vi "Finish.vi"   [LabVIEW 2014]
doc: "This VI is called just before exiting. It is expected to close I/O refnum, save collected data, etc."
uses:
  <vilib>/Rock Robotics/WPI/Joystick/WPI_JoystickGetSetRefNum.vi
  <vilib>/Rock Robotics/WPI/RobotDrive/WPI_RobotDriveGetSetRefNum.vi
types:
  T1 = typedef "WPI_JoystickDevRef.ctl" = cluster{"Device":T2}
  T2 = typedef "WPI_JoystickDeviceEnum.ctl" = enum16{"USB 0", "USB 1", "USB 2", "USB 3", "USB 4", "USB 5"}
  T3 = typedef "WPI_RobotDriveDevRef.ctl" = cluster{"DevStatus":errorcluster, "Motors[]":T4[], "Square Inputs":bool, "Max Output":dbl}
  T4 = typedef "WPI_MotorControlDeviceRef.ctl" = cluster{"DeviceStatus":errorcluster, "Type":T5, "PWM":cluster{"Controller":T6, "PWM Channel":T7, "DeadBand":T8}, "CAN":cluster{"Device Number":u8, "Control Mode":T9, "Semaphore":T10, "Max Vout":dbl, "TalonSRX Control Mode":T11}, "Invert":bool, "TransformRef":T12, "InvTransformRef":T12}
  T5 = typedef "WPI_MotorControlType.ctl" = enum16{"PWM", "CAN", "CANTalonSRX"}
  T6 = typedef "FPGA_TypedefDigitalModule.ctl" = enum16{"Controller 1"}
  T7 = typedef "FPGA_DIOPWMChannel.ctl" = enum8{"PWM 0", "PWM 1", "PWM 2", "PWM 3", "PWM 4", "PWM 5", "PWM 6", "PWM 7", "PWM 8", "PWM 9", "PWM MXP 0", "PWM MXP 1", "PWM MXP 2", "PWM MXP 3", "PWM MXP 4", "PWM MXP 5", "PWM MXP 6", "PWM MXP 7", "PWM MXP 8", "PWM MXP 9", "Invalid"}
  T8 = typedef "WPI_PWMDeadband.ctl" = cluster{"Name":string, "maxPositivePwm":i32, "minPositivePwm":i32, "centerPwm":i32, "maxNegativePwm":i32, "minNegativePwm":i32, "angularRange":u16}
  T9 = typedef "WPI_CANJaguar_ControlMode.ctl" = enum8{"Percent VBus", "Current", "Speed", "Position", "Voltage"}
  T10 = typedef "Semaphore RefNum" = refnum<k1>
  T11 = typedef "WPI_CANTalonSRX_APIControlMode.ctl" = enum8{"Percent VBus", "Speed", "Position", "Slave", "Unchanged / Invalid"}
  T12 = typedef "WPI_PWMTransform_ConPane.ctl" = refnum<vi>
  T13 = typedef "WPI_SolenoidDevRef.ctl" = cluster{"DevStatus":errorcluster, "Pneumatics Control Module":u8, "Forward Solenoid Channel":T14, "Reverse Solenoid Channel":T14}
  T14 = typedef "WPI_SolenoidChannel.ctl" = enum8{"Solenoid 0", "Solenoid 1", "Solenoid 2", "Solenoid 3", "Solenoid 4", "Solenoid 5", "Solenoid 6", "Solenoid 7", "Invalid"}
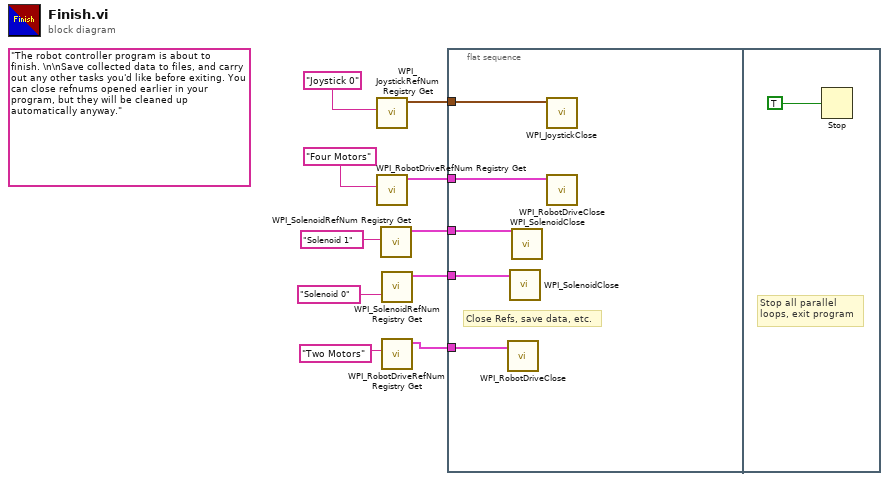
[diagram p0: block diagram]
diagram:
  (unwired) "The robot controller program is about to finish. \n\nSave collected data to files, and carry out any other tasks you'd like before exiting. You can close refnums opened earlier in your program, but they will be cleaned up automatically anyway."
  n1 = call <vilib>:"WPI_JoystickRefNum Registry Get.vi"("refnum name"="Joystick 0") -> ("JoystickDevRef"=w7:T1)  [unwired: 1 in, 9 out]
  n2 = call <vilib>:"WPI_RobotDriveRefNum Registry Get.vi"("refnum name"="Four Motors") -> ("RobotDriveDevRef"=w8:T3)  [unwired: 1 in, 9 out]
  n3 = call <vilib>:"WPI_SolenoidRefNum Registry Get.vi"("refnum name"="Solenoid 1") -> ("SolenoidDevRef"=w5:T13)  [unwired: 9 in, 1 out]
  n4 = call <vilib>:"WPI_SolenoidRefNum Registry Get.vi"("refnum name"="Solenoid 0") -> ("SolenoidDevRef"=w3:T13)  [unwired: 9 in, 1 out]
  n5 = call <vilib>:"WPI_RobotDriveRefNum Registry Get.vi"("refnum name"="Two Motors") -> ("RobotDriveDevRef"=w2:T3)  [unwired: 9 in, 1 out]
  n6 = flat-sequence {
    tunnel: w8 -> [w15]
    tunnel: w7 -> [w14]
    tunnel: w5 -> [w13]
    tunnel: w3 -> [w12]
    tunnel: w2 -> [w11]
    frame #0 {
      # "Close Refs, save data, etc."
      n7 = call <vilib>:"WPI_RobotDriveClose.vi"("RobotDriveDevRef"=w11) -> ()  [unwired: 10 in, 1 out]
      n8 = call <vilib>:"WPI_SolenoidClose.vi"("SolenoidDevRef"=w12) -> ()  [unwired: 10 in, 1 out]
      n9 = call <vilib>:"WPI_SolenoidClose.vi"("SolenoidDevRef"=w13) -> ()  [unwired: 10 in, 1 out]
      n10 = call <vilib>:"WPI_JoystickClose.vi"("JoystickDevRef"=w14) -> ()  [unwired: 11 out]
      n11 = call <vilib>:"WPI_RobotDriveClose.vi"("RobotDriveDevRef"=w15) -> ()  [unwired: 1 in, 10 out]
    }
    frame #1 {
      # "Stop all parallel\nloops, exit program"
      n12 = Stop(stop? (T)=TRUE ("Quit")) -> ()
    }
  }
